vi "test.vi"   [LabVIEW 2012]
uses:
  Chat/Chat.lvclass
  <vilib>/Distrio/Murmex/Murmex/Murmex.lvclass
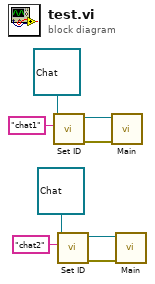
[diagram p0: block diagram]
diagram:
  n1 = call <vilib>:"Set ID.vi"("id"="chat1", "Murmex in"=refnum<class "Chat.lvclass"> refnum ("Chat")) -> ("error out"=w7:errorcluster, "Murmex out"=w8:refnum<class "Chat.lvclass">)  [unwired: 8 in]
  n2 = call <vilib>:"Set ID.vi"("id"="chat2", "Murmex in"=refnum<class "Chat.lvclass"> refnum ("Chat")) -> ("error out"=w2:errorcluster, "Murmex out"=w1:refnum<class "Chat.lvclass">)  [unwired: 8 in]
  n3 = call-dynamic "Main.vi"("error in (no error)"=w7, "ChatBase in"=w8) -> ()  [unwired: 8 in, 2 out]
  n4 = call-dynamic "Main.vi"("error in (no error)"=w2, "ChatBase in"=w1) -> ()  [unwired: 8 in, 2 out]
